vi "2206273_Two_Edge_Separation.vi"() -> ()   [LabVIEW 2014]
doc: "I. Description:\nThis example demonstrates how to perform a two edge separation measurement on a Counter Input Channel. The First Edge, Second Edge, Minimum Value, and Maximum Value are all configurable. \n\nThis example shows how to perform a two edge separation measurement on the counter's default input terminals (refer to section IV, I/O Connections Overview, below for more information), but could easily be expanded to measure two edge separation on any PFI, RTSI, or internal signal.\n\nRefer to your device documentation to see if your device supports two edge separation measurements.\n\nII. Instructions for Running:\n1. Select the Physical Channel which corresponds to the counter on the DAQ device you want to perform a two edge separation measurement on.\n2. Enter the First Edge and Second Edge corresponding to the two edges you want the counter to measure. Enter the Maximum and Minimum Value to specify the range of your unknown two edge separation. Additionally, you can change the First and Second Edge Input Terminals using the channel property node.\nNote: It is important to set the Maximum and Minimum Values of your unknown two edge separation as accurately as possible so the best internal timebase can be chosen to minimize measurement error. The default values specify a range that can be measured by the counter using the 20MHzTimebase.\n\nIII. Block Diagram Steps:\n1. Create a Counter Input channel to perform a Two Edge Separation measurement. The First and Second Edge parameters are used to specify the rising or falling edge of one digital signal and the rising or falling edge of another digital signal. It is important to set the Maximum and Minimum Values of your unknown two edge separation as accurately as possible so the best internal timebase can be chosen to minimize measurement error. The default values specify a range that can be measured by the counter using the 20MHzTimebase.\n2. Call the Read VI to return the next two edge separation measurement. Set a timeout so an error is returned if an edge separation is not returned in the specified time limit.\n3. Call the Clear Task VI to clear the Task \n4. Use the popup dialog box to display an error if any.\n\nIV. I/O Connections Overview:\nThe counter will perform a two edge separation measurement on the First and Second Edge Input Terminals of the counter specified in the Physical Channel I/O control. \n\n In this example the two edge separation will be measured on the default input terminals on ctr0. \n\nFor more information on the default counter input and output terminals for your device, open the NI-DAQmx Help, and refer to Counter Signal Connections found under the Device Considerations book in the table of contents."
uses:
  <vilib>/Utility/error.llb/DialogType.ctl
  <vilib>/DAQmx/create/channels.llb/DAQmx Create Channel (CI-Two Edge Separation).vi
  <vilib>/DAQmx/read.llb/DAQmx Read (Counter DBL 1Chan 1Samp).vi
panel:
  out "ctr2 task":refnum<k21>
  out "ctr1 task":refnum<k21>
  in  "Tab Control":enum32{"SYSTEM", "MEASURE"}(tab)=enum."MEASURE"
  in  "Physical Channel":tag="LightScreens/ctr0" caption="Physical Channel 1"
  in  "Minimum Value (sec)":dbl=1e-07 format="%0.9f"
  in  "Maximum Value (sec)":dbl=0.05 format="%0.9f"
  in  "First Edge":i32(ring)=10280 items=["Rising"=10280, "Falling"=10171]
  in  "Second Edge":i32(ring)=10280 items=["Rising"=10280, "Falling"=10171]
  in  "Second Edge 2":i32(ring)=10280 items=["Rising"=10280, "Falling"=10171]
  in  "First Edge 2":i32(ring)=10280 items=["Rising"=10280, "Falling"=10171]
  in  "Maximum Value (sec) 2":dbl=0.05 caption="Maximum Value (sec)" format="%0.9f"
  in  "Minimum Value (sec) 2":dbl=1e-07 caption="Minimum Value (sec)" format="%0.9f"
  in  "Physical Channel 2":tag="LightScreens/ctr1"
  out "armed":bool
  out "Measured Two Edge Separation (sec)":dbl caption="1 -  Measured Two Edge Separation (sec)" format="%0.9f"
  in  "Take measurement":bool
  out "Measured Two Edge Separation (sec) 2":dbl caption="2 - Measured Two Edge Separation (sec)" format="%0.9f"
  in  "stop":bool
  # "Channel Parameters"
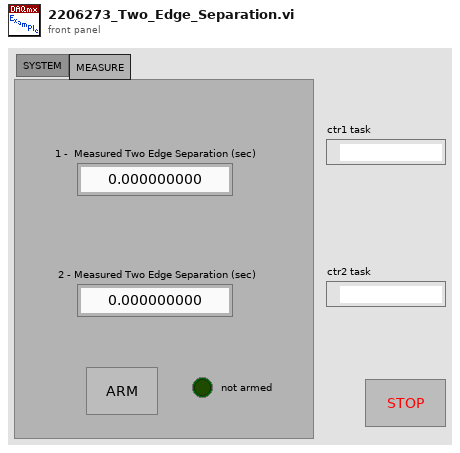
[diagram p1: front panel]
types:
  T1 = typedef "DialogType.ctl" = u16
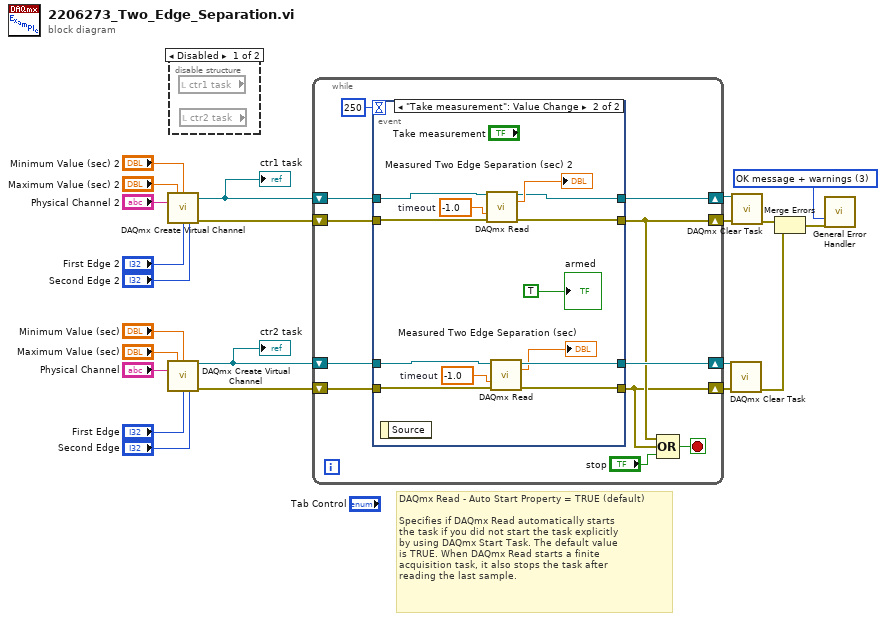
[diagram p0: block diagram]
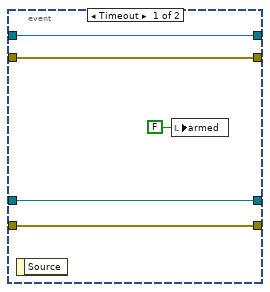
[diagram p3: hidden frame]
diagram:
  w19 = T1 3 items=["no dialog", "OK message", "continue or stop message", "OK message + warnings", "continue/stop + warnings"] ("type of dialog (OK msg:1)")
  # "DAQmx Read - Auto Start Property = TRUE (default)\n\nSpecifies if DAQmx Read automatically starts \nthe task if you did not start the task explicitly \nby using DAQmx Start Task. The default value \nis TRUE. When DAQmx Read starts a finite \nacquisition task, it also stops the task after \nreading the last sample."
  n1 = call-poly <vilib>:"DAQmx Create Virtual Channel.vi"("maximum value"="Maximum Value (sec) 2", "minimum value"="Minimum Value (sec) 2", "counter"="Physical Channel 2", "first edge"="First Edge 2", "second edge"="Second Edge 2") -> ("task out"=w4:refnum<k21>, "error out"=w1:errorcluster)  [unwired: 9 in]
  "ctr1 task" <- w4
  n2 = call-poly <vilib>:"DAQmx Create Virtual Channel.vi"("maximum value"="Maximum Value (sec)", "minimum value"="Minimum Value (sec)", "counter"="Physical Channel", "first edge"="First Edge", "second edge"="Second Edge") -> ("task out"=w3:refnum<k21>, "error out"=w2:errorcluster)  [unwired: 9 in]
  "ctr2 task" <- w3
  n3 = disable-structure shown="Disabled" {
    frame Disabled {
      n4 = local read "ctr1 task"() -> ()  [unwired: 1 out]
      n5 = local read "ctr2 task"() -> ()  [unwired: 1 out]
    }
    frame Enabled {
    }
  }
  n6 = while {
    shift-right: [w31] -> w15
    shift-left: w3 -> [w33]
    shift-right: [w25] -> w16
    shift-left: w2 -> [w32]
    shift-right: [w29] -> w14
    shift-left: w4 -> [w27]
    shift-right: [w26] -> w13
    shift-left: w1 -> [w28]
    stop <- w23 stop-if-true
    n7 = event shown="[1] \"Take measurement\": Value Change" {
      selector: _ -> [_ _]
      dyn-events: _ -> [_ _]
      timeout: 250 -> [_ _]
      tunnel: w33 -> [w36 w39]
      tunnel: w32 -> [w35 w50]
      tunnel: [w35 w49] -> w25
      tunnel: [w36 w48] -> w31
      tunnel: w27 -> [w38 w40]
      tunnel: w28 -> [w37 w43]
      tunnel: [w37 w44] -> w26
      tunnel: [w38 w45] -> w29
      event Timeout {
        n8 = event-data() -> ()  [unwired: 1 in, 1 out]
        n9 = local write "armed"(FALSE ("armed")) -> ()
      }
      event "Take measurement": Value Change {
        w42 = -1.0  # timeout
        w51 = -1.0  # timeout
        n10 = event-data() -> ()  [unwired: 1 in, 1 out]
        n11 = call-poly <vilib>:"DAQmx Read.vi"("task/channels in"=w40, "timeout"=w42, "error in"=w43) -> ("task out"=w45:refnum<k21>, "data"=→"Measured Two Edge Separation (sec) 2":dbl, "error out"=w44:errorcluster)  [unwired: 10 in]
        n12 = call-poly <vilib>:"DAQmx Read.vi"("task/channels in"=w39, "timeout"=w51, "error in"=w50) -> ("task out"=w48:refnum<k21>, "data"=→"Measured Two Edge Separation (sec)":dbl, "error out"=w49:errorcluster)  [unwired: 10 in]
        "armed" <- TRUE ("armed")
      }
    }
    n13 = Compound Arithmetic op=OR(w26, w25, "stop") -> (w23:bool)
  }
  n14 = call <vilib>:"DAQmx Clear Task.vi"("task in"=w15, "error in"=w16) -> ("error out"=w7:errorcluster)  [unwired: 13 in]
  n15 = call <vilib>:"DAQmx Clear Task.vi"("task in"=w14, "error in"=w13) -> ("error out"=w6:errorcluster)  [unwired: 13 in]
  n16 = Merge Errors(w6, w7) -> (w5:errorcluster)
  n17 = call <vilib>:"General Error Handler.vi"("type of dialog (OK msg:1)"=w19, "error in (no error)"=w5) -> ()  [unwired: 9 in, 5 out]
